vi "picoSetMem.vi"(8 "error in (no error)":errorcluster, 10 "Rapid Block Acquisition Settings":T1={"preTriggerSamples"=0, "postTriggerSamples"=1000, "timebase"=2, "Down-Sample Mode"=0, "Down Sample Ratio"=1, "Oversample"=1, "Number of Captures"=10} {"Down Sample Ratio" min=1 step=1; "Down-Sample Mode" items=["None"=0, "Aggregate"=1, "Decimate"=2, "Average"=4]}, 11 "Handle In":i16) -> (0 "error out":errorcluster, 1 "timebase":u32, 2 "postTriggerSamples":u32, 3 "Handle Out":i16, 5 "nCaptures":u16)   [LabVIEW 2011]
uses:
  PS2000a.dll
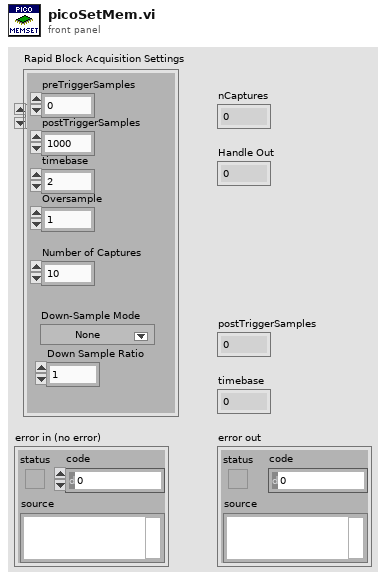
[diagram p1: front panel]
types:
  T1 = cluster{"preTriggerSamples":u32, "postTriggerSamples":u32, "timebase":u32, "Down-Sample Mode":i32, "Down Sample Ratio":u32, "Oversample":i16, "Number of Captures":u32}
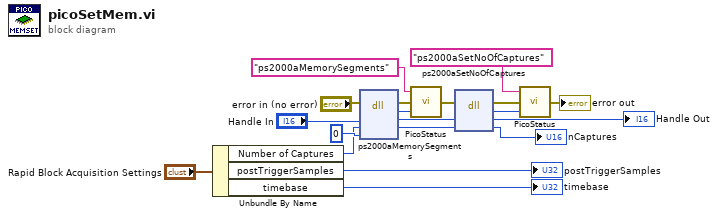
[diagram p0: block diagram]
diagram:
  n1 = Unbundle By Name("Rapid Block Acquisition Settings") -> ("Number of Captures"=w2:u32, "postTriggerSamples"=→"postTriggerSamples":u32, "timebase"=→"timebase":u32)
  n2 = dll-call lib="ps2000a.dll" fn="ps2000aMemorySegments" ("ps3000.dll:_ps3000_open_unit@0")(error in="error in (no error)", "handle"="Handle In", "nSegments"=w2, "nMaxSamples"=u32 0) -> (error out=w6:errorcluster, "PICO_STATUS"=w5:i32, "handle"=w10:i16, "nSegments"=w9:u32)  [unwired: 3 in, 1 out]
  n3 = call "PicoStatus.vi"("PICO STATUS"=w5, "error in"=w6, "source"="ps2000aMemorySegments") -> ("error out"=w11:errorcluster)
  n4 = dll-call lib="ps2000a.dll" fn="ps2000aSetNoOfCaptures" ("ps3000.dll:_ps3000_open_unit@0")(error in=w11, "handle"=w10, "nCaptures"=w9) -> (error out=w13:errorcluster, "PICO_STATUS"=w12:i32, "handle"=→"Handle Out":i16, "nCaptures"=→"nCaptures":u16)  [unwired: 2 in, 1 out]
  n5 = call "PicoStatus.vi"("PICO STATUS"=w12, "error in"=w13, "source"="ps2000aSetNoOfCaptures") -> ("error out"=→"error out":errorcluster)
